vi "Must Call Child Method.vi"(8 "error in":errorcluster) -> (0 "error out":errorcluster)   [LabVIEW 2020]
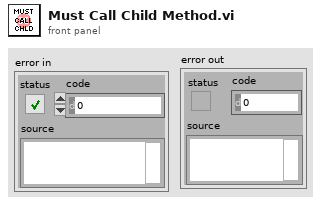
[diagram p1: front panel]
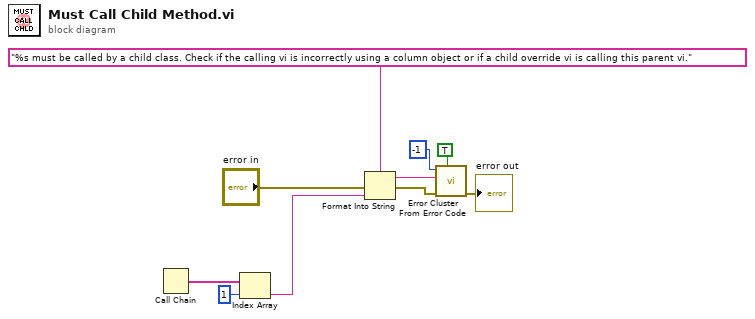
[diagram p0: block diagram]
diagram:
  n1 = Call Chain() -> (call chain=w3:string[])
  n2 = Index Array(array=w3, index=1) -> (element=w1:string)
  n3 = Format Into String(format string="%s must be called by a child class. Check if the calling vi is incorrectly using a column object or if a child override vi is calling this parent vi.", error in="error in", w1) -> (resulting string=w7:string, error out=w6:errorcluster)  [unwired: 1 in]
  n4 = call <vilib>:"Error Cluster From Error Code.vi"("show call chain? (False)"=TRUE, "error in (no error)"=w6, "error message (\"\")"=w7, "error code (0)"=-1) -> ("error out"=→"error out":errorcluster)  [unwired: 5 in]
